vi "Initialization.vi"(7 "CostFunction":refnum<vi>, 8 "Error In":errorcluster, 10 "CostFunctionData":variant, 11 "basic_config":T2) -> (0 "Error Out":errorcluster, 3 "GenAlg_data":T1)   [LabVIEW 2016]
uses:
  TypeDefs/basic_config.ctl
  TypeDefs/GenAlg_data.ctl
  TypeDefs/element.ctl
  TypeDefs/geration_data.ctl
  TypeDefs/selection_data.ctl
  TypeDefs/SimulatedAnnealing_data.ctl
  TypeDefs/multi_eval_data.ctl
  TypeDefs/termination_data.ctl
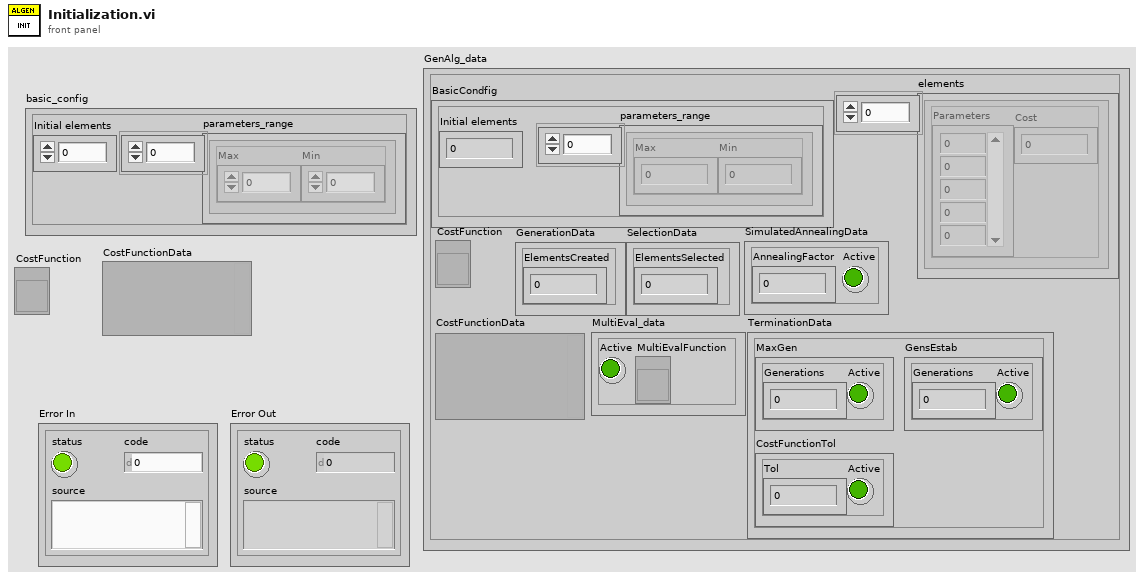
[diagram p1: front panel]
types:
  T1 = typedef "GenAlg_data.ctl" = cluster{"BasicCondfig":T2, "elements":T3[], "CostFunction":refnum<vi>, "GenerationData":T4, "SelectionData":T5, "SimulatedAnnealingData":T6, "CostFunctionData":variant, "MultiEval_data":T7, "TerminationData":T8}
  T2 = typedef "basic_config.ctl" = cluster{"parameters_range":cluster{"Max":dbl, "Min":dbl}[], "Initial elements":i32}
  T3 = typedef "element.ctl" = cluster{"Parameters":dbl[], "Cost":dbl}
  T4 = typedef "geration_data.ctl" = cluster{"ElementsCreated":i32}
  T5 = typedef "selection_data.ctl" = cluster{"ElementsSelected":i32}
  T6 = typedef "SimulatedAnnealing_data.ctl" = cluster{"AnnealingFactor":dbl, "Active":bool}
  T7 = typedef "multi_eval_data.ctl" = cluster{"Active":bool, "MultiEvalFunction":refnum<vi>}
  T8 = typedef "termination_data.ctl" = cluster{"MaxGen":cluster{"Generations":i32, "Active":bool}, "CostFunctionTol":cluster{"Tol":dbl, "Active":bool}, "GensEstab":cluster{"Generations":i32, "Active":bool}}
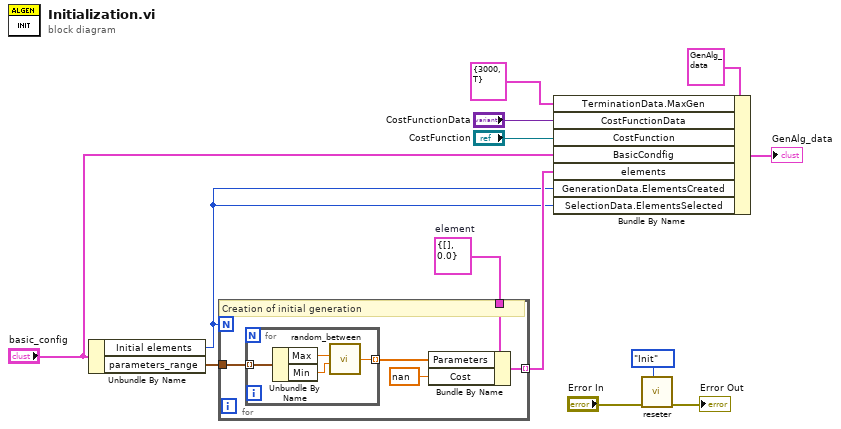
[diagram p0: block diagram]
diagram:
  w8 = T3 {"Parameters"=[], "Cost"=0.0}  # element
  n1 = Unbundle By Name("basic_config") -> ("Initial elements"=w7:i32, "parameters_range"=w13:cluster{"Max":dbl, "Min":dbl}[])
  n2 = for {
    N: w7 -> [_]
    tunnel: w13 -> [w18]
    tunnel: [w16] -> w10 mode=indexing
    tunnel: w8 -> [w15]
    # "Creation of initial generation"
    n3 = for {
      tunnel: w18 -> [w22] mode=indexing
      tunnel: [w19] -> w17 mode=indexing
      n4 = Unbundle By Name(w22) -> ("Max"=w21:dbl, "Min"=w20:dbl)
      n5 = call "random_between.vi"("b"=w20, "a"=w21) -> ("Random"=w19:dbl)  [unwired: 4 in]
    }
    n6 = Bundle By Name(cluster=w15, "Parameters"=w17, "Cost"=nan) -> (w16:T3)
  }
  n7 = Bundle By Name(cluster=T1 {"BasicCondfig"={"parameters_range"=[], "Initial elements"=0}, "elements"=[], "CostFunction"=refnum, "GenerationData"={"ElementsCreated"=0}, "SelectionData"={"ElementsSelected"=0}, "SimulatedAnnealingData"={"AnnealingFactor"=0.0, "Active"=FALSE}, "CostFunctionData"=variant, "MultiEval_data"={"Active"=FALSE, "MultiEvalFunction"=refnum}, "TerminationData"={"MaxGen"={"Generations"=0, "Active"=FALSE}, "CostFunctionTol"={"Tol"=0.0, "Active"=FALSE}, "GensEstab"={"Generations"=0, "Active"=FALSE}}} ("GenAlg_data"), "TerminationData.MaxGen"=cluster{"Generations":i32, "Active":bool} {"Generations"=3000, "Active"=TRUE}, "CostFunctionData"="CostFunctionData", "CostFunction"="CostFunction", "BasicCondfig"="basic_config", "elements"=w10, "GenerationData.ElementsCreated"=w7, "SelectionData.ElementsSelected"=w7) -> (→"GenAlg_data":T1)
  n8 = call "reseter.vi"("Mode"=enum16{"Init", "Set", "Get"}."Init", "Error In"="Error In") -> ("Error Out"=→"Error Out":errorcluster)  [unwired: 8 in, 1 out]
